vi "k2182_timer_buffer-read.vi"() -> ()   [LabVIEW 2022 SP3]
uses:
  <instrlib>/Keithley 2182/Keithley 2182.lvlib
panel:
  out "Waveform Graph":dbl[](graph)
  out "error out":errorcluster
  in  "Autorange":bool=TRUE
  in  "Masurement Range":dbl=10.0
  in  "Voltage Resolution":i32=8
  in  "Integration Rate Units":i32(ring) items=["Line Cycles", "Seconds"]
  in  "Integration Rate":dbl=5.0
  in  "Measurement":i32(ring) items=["Voltage Channel 1", "Voltage Channel 2", "Temperature Channel 1", "Temperature Channel 2"]
  in  "Buffer Source":i32(ring)=1 items=["None", "Measurements", "Math Calculation"]
  in  "Measurements/Buffer Size":i32=10 min=2 max=1024 step=1
  out "Buffer Metadata":T1(array[cluster])
  out "Buffer":dbl[](array[numeric])
  out "Mean":dbl=1.0
  out "Maximum":dbl
  out "Standard Deviation":dbl
  out "Minimum":dbl
  in  "Autodelay (T: Enable)":bool=TRUE
  in  "Trigger Delay (s)":dbl
  in  "Timer Interval (s)":dbl=0.1 format="%#_13g"
  in  "VISA resource name":refnum<visa-resource-name>
  # "Keithley 2182 - Voltage Reading using timer"
  # "Measurement Settings"
  # "Data Buffer Readings"
  # "Trigger Timer Settings"
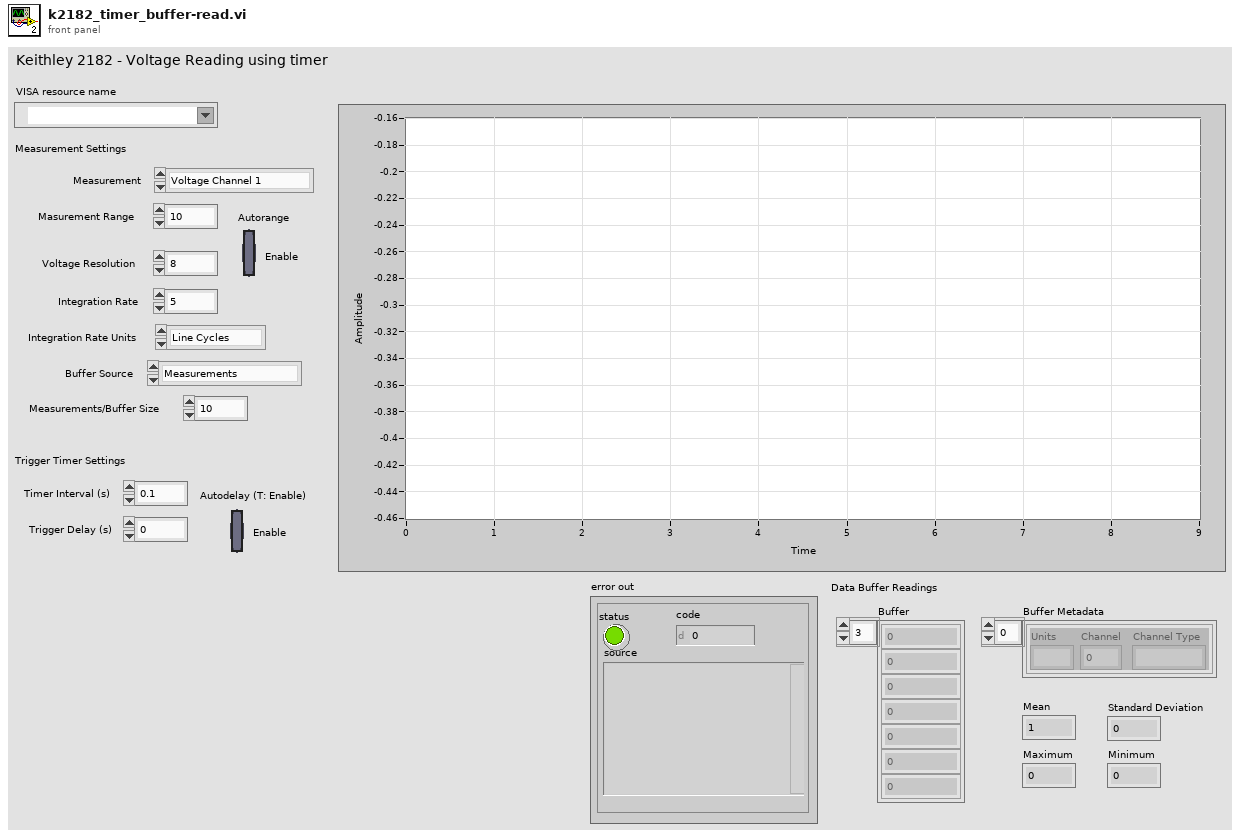
[diagram p1: front panel]
types:
  T1 = cluster{"Units":string, "Channel":i32, "Channel Type":string}[]
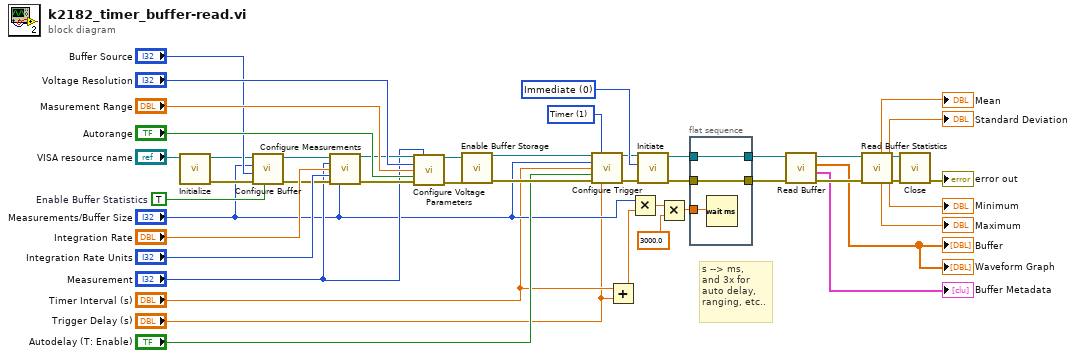
[diagram p0: block diagram]
diagram:
  w10 = 1 items=["Immediate", "Timer", "Manual", "Bus", "External"] ("Trigger Source (0: Immediate)")
  w17 = 0 items=["Immediate", "Continuous"] ("Initiate Type (0: Immediate)")
  w32 = TRUE  # Enable Buffer Statistics
  # "s --> ms, \nand 3x for\nauto delay, \nranging, etc.."
  n1 = call <instrlib>:"Initialize.vi"("VISA resource name"="VISA resource name") -> ("error out"=w35:errorcluster, "VISA resource name out"=w34:refnum<visa-resource-name>)  [unwired: 9 in]
  n2 = call <instrlib>:"Configure Buffer.vi"("Enable Buffer Statistics (0: Disable)"=w32, "error in (no error)"=w35, "Buffer Source (0: None)"="Buffer Source", "Buffer Size (2)"="Measurements/Buffer Size", "VISA resource name"=w34) -> ("error out"=w43:errorcluster, "VISA resource name out"=w42:refnum<visa-resource-name>)  [unwired: 5 in]
  n3 = call <instrlib>:"Configure Measurements.vi"("VISA resource name"=w42, "Measurement (0: Voltage Channel 1)"="Measurement", "Integration Rate (5)"="Integration Rate", "Integration Rate Units (0: Line Cycles)"="Integration Rate Units", "error in (no error)"=w43, "Sample Count (1)"="Measurements/Buffer Size") -> ("VISA resource name out"=w37:refnum<visa-resource-name>, "error out"=w38:errorcluster)  [unwired: 8 in]
  n4 = call <instrlib>:"Configure Voltage Parameters.vi"("VISA resource name"=w37, "Measurement (1: Voltage Channel 1)"="Measurement", "Voltage Resolution (8)"="Voltage Resolution", "Range Value (12)"="Masurement Range", "Autorange (T: Enable)"="Autorange", "error in (no error)"=w38) -> ("VISA resource name out"=w15:refnum<visa-resource-name>, "error out"=w16:errorcluster)  [unwired: 8 in]
  n5 = call <instrlib>:"Enable Buffer Storage.vi"("error in (no error)"=w16, "VISA resource name"=w15) -> ("error out"=w13:errorcluster, "VISA resource name out"=w14:refnum<visa-resource-name>)  [unwired: 8 in]
  n6 = call "Configure Trigger.vi"("VISA resource name"=w14, "Trigger Source (0: Immediate)"=w10, "Trigger Count (1)"="Measurements/Buffer Size", "Timer Interval (0.1 s)"="Timer Interval (s)", "Autodelay (T: Enable)"="Autodelay (T: Enable)", "error in (no error)"=w13, "Trigger Delay (0 s)"="Trigger Delay (s)") -> ("VISA resource name out"=w11:refnum<visa-resource-name>, "error out"=w12:errorcluster)  [unwired: 7 in]
  n7 = Add(x="Timer Interval (s)", y="Trigger Delay (s)") -> (x+y=w4:dbl)
  n8 = Multiply(x="Measurements/Buffer Size", y=w4) -> (x*y=w8:dbl)
  n9 = call <instrlib>:"Initiate.vi"("error in (no error)"=w12, "Initiate Type (0: Immediate)"=w17, "VISA resource name"=w11) -> ("error out"=w23:errorcluster, "VISA resource name out"=w21:refnum<visa-resource-name>)  [unwired: 7 in]
  n10 = Multiply(x=w8, y=3000.0) -> (x*y=w3:dbl)
  n11 = flat-sequence {
    tunnel: w3 -> [w49]
    tunnel: [w48] -> w24
    tunnel: w23 -> [w48]
    tunnel: [w47] -> w22
    tunnel: w21 -> [w47]
    frame #0 {
      n12 = Wait (ms)(milliseconds to wait=w49) -> ()  [unwired: 1 out]
    }
  }
  n13 = call <instrlib>:"Read Buffer.vi"("error in (no error)"=w24, "VISA resource name"=w22) -> ("error out"=w31:errorcluster, "Buffer Metadata"=→"Buffer Metadata":T1, "Buffer"=→"Buffer" →"Waveform Graph":dbl[], "VISA resource name out"=w30:refnum<visa-resource-name>)  [unwired: 6 in]
  n14 = call <instrlib>:"Read Buffer Statistics.vi"("error in (no error)"=w31, "VISA resource name"=w30) -> ("error out"=w20:errorcluster, "Minimum"=→"Minimum":dbl, "Standard Deviation"=→"Standard Deviation":dbl, "VISA resource name out"=w19:refnum<visa-resource-name>, "Maximum"=→"Maximum":dbl, "Mean"=→"Mean":dbl)  [unwired: 4 in]
  n15 = call <instrlib>:"Close.vi"("error in (no error)"=w20, "VISA resource name"=w19) -> ("error out"=→"error out":errorcluster)  [unwired: 9 in]
